vi "Encoder_PanelSim_Global.vi"(0 "menu":T5=enum."set reset", 5 "EncoderIndex":T4, 7 "Value Set":bool, 9 "Numeric Value":dbl format="%#.4f", 11 "error in (no error)":errorcluster, 12 "String Value":string, 13 "Values":T1) -> (10 "Encoder new":T2={"type"="Encoder", "device"="", "name"="", "data"={"<init"=FALSE, ">count"=0.0, ">period"=0.0, "<samples_to_avg"=0, "<offset"=0.0, "<channel_a"=0, "<channel_b"=0}}, 15 "error out":errorcluster)   [LabVIEW 2019]
doc: "This is used to set and get the last motor output values. This is needed for simulation, since we cannot read these values from the hardware.\n\nThis software is licensed. Open the labview\\readme\\WPI Robotics Library Open Source License.txt file for more information."
uses:
  Encoder Update Ops.ctl
  Encoder proto.ctl
  Encoder data protoo.ctl
  <vilib>/Rock Robotics/SystemInterfaces/Encoder/FPGA_EncoderIdx.ctl
  Encoder Values.ctl
panel:
  out "All Values":T2[](array[typedef])
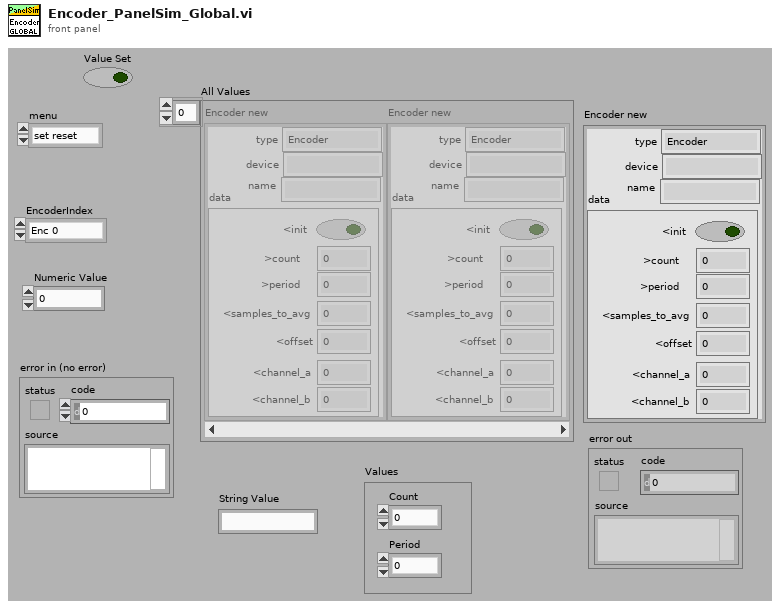
[diagram p1: front panel]
types:
  T1 = typedef "Encoder Values.ctl" = cluster{"Count":dbl, "Period":dbl}
  T2 = typedef "Encoder proto.ctl" = cluster{"type":string, "device":string, "name":string, "data":T3}
  T3 = typedef "Encoder data protoo.ctl" = cluster{"<init":bool, ">count":dbl, ">period":dbl, "<samples_to_avg":i32, "<offset":dbl, "<channel_a":i32, "<channel_b":i32}
  T4 = typedef "FPGA_EncoderIdx.ctl" = enum8{"Enc 0", "Enc 1", "Enc 2", "Enc 3", "Enc 4", "Enc 5", "Enc 6", "Enc 7", "Invalid"}
  T5 = typedef "Encoder Update Ops.ctl" = enum16{"set init", "set count", "set period", "set reset", "set samples_to_avg", "get", "delete", "JSON update", "set name", "transmit initial", "reset", "set channel_a", "set channel_b", "set values"}
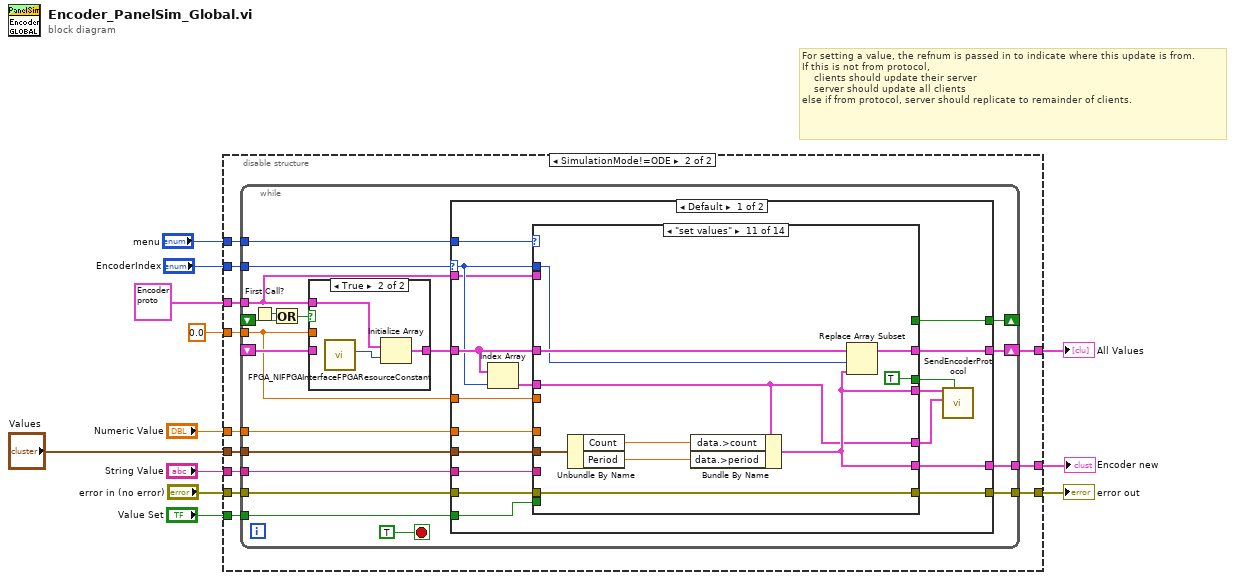
[diagram p0: block diagram]
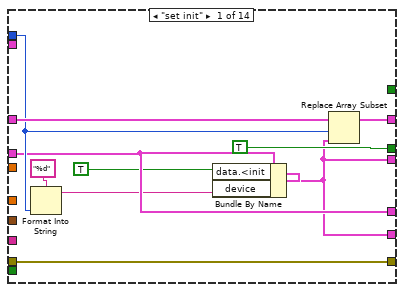
[diagram p3: hidden frame]
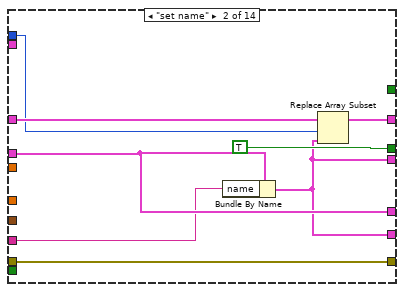
[diagram p4: hidden frame]
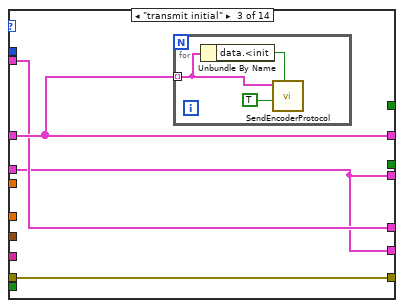
[diagram p5: hidden frame]
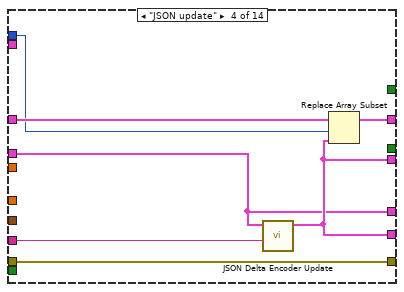
[diagram p6: hidden frame]
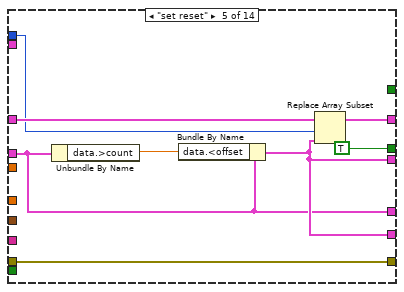
[diagram p7: hidden frame]
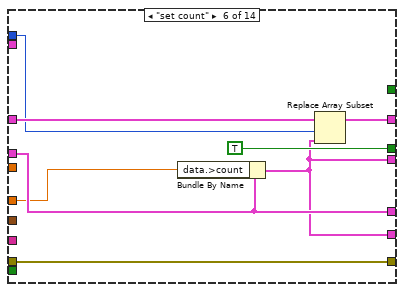
[diagram p8: hidden frame]
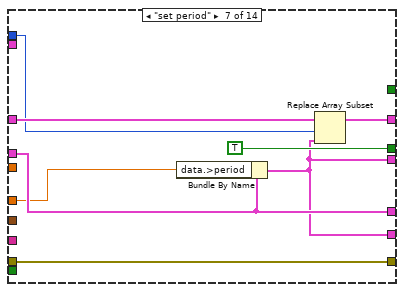
[diagram p9: hidden frame]
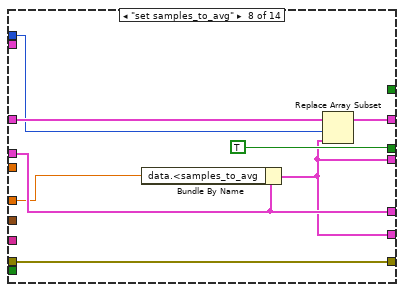
[diagram p10: hidden frame]
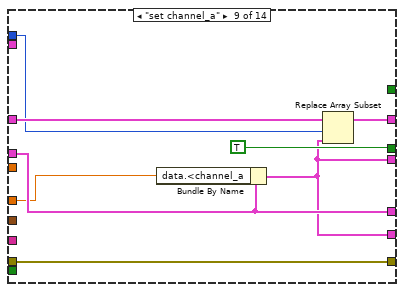
[diagram p11: hidden frame]
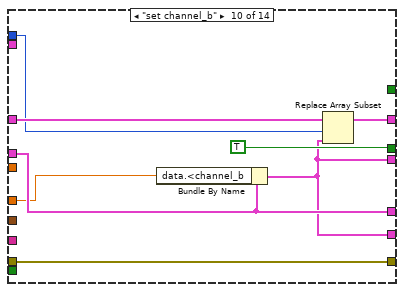
[diagram p12: hidden frame]
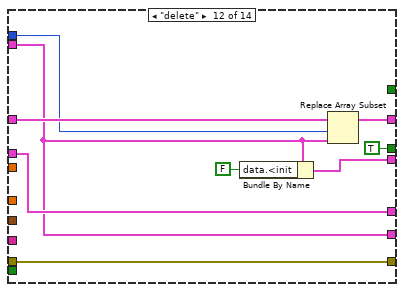
[diagram p13: hidden frame]
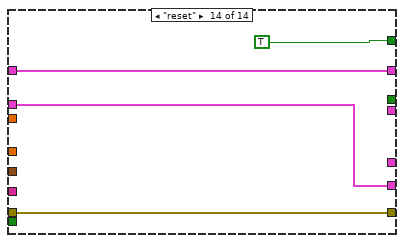
[diagram p15: hidden frame]
diagram:
  # "For setting a value, the refnum is passed in to indicate where this update is from.\nIf this is not from protocol,\n    clients should update their server\n    server should update all clients\nelse if from protocol, server should replicate to remainder of clients."
  n1 = disable-structure shown="SimulationMode!=ODE" {
    disable-tunnel: "menu" -> [_ w26]
    disable-tunnel: [w14 w25] -> w11
    disable-tunnel: "error in (no error)" -> [w14 w24]
    disable-tunnel: [_ w23] -> w9
    disable-tunnel: 0.0 ("Output") -> [_ w22]
    disable-tunnel: "EncoderIndex" -> [_ w21]
    disable-tunnel: [w13 w20] -> w6
    disable-tunnel: T2 {"type"="Encoder", "device"="", "name"="", "data"={"<init"=FALSE, ">count"=0.0, ">period"=0.0, "<samples_to_avg"=0, "<offset"=0.0, "<channel_a"=0, "<channel_b"=0}} ("Encoder new") -> [w13 w19]
    disable-tunnel: "String Value" -> [_ w18]
    disable-tunnel: "Numeric Value" -> [_ w17]
    disable-tunnel: "Value Set" -> [_ w16]
    disable-tunnel: "Values" -> [_ w15]
    frame condition #0 {
    }
    frame condition #1 (active) {
      n2 = while {
        tunnel: w24 -> [w42]
        shift-right: [w45] -> w23
        shift-left: _ -> [w38]
        tunnel: [w44] -> w20
        tunnel: w26 -> [w43]
        tunnel: [w41] -> w25
        tunnel: w21 -> [w36]
        tunnel: w22 -> [w37]
        tunnel: w19 -> [w35]
        tunnel: w18 -> [w34]
        tunnel: w17 -> [w33]
        tunnel: w16 -> [w32]
        shift-right: [w28] -> _
        shift-left: _ -> [w29]
        tunnel: w15 -> [w27]
        stop <- TRUE stop-if-true
        n3 = First Call?() -> (First Call?: T/F=w31:bool)
        n4 = Or(x=w31, y=w29) -> (x .or. y?=w30:bool)
        n5 = case shown="True" w30 {
          tunnel: [w173 w176] -> w39
          tunnel: w38 -> [w173 _]
          tunnel: w37 -> [_ _]
          tunnel: w35 -> [_ w175]
          frame False {
          }
          frame True {
            n6 = call <vilib>:"FPGA_NIFPGAInterfaceFPGAResourceConstant.vi"() -> ("NumberOfEncoders"=w174:u32)  [unwired: 11 out]
            n7 = Initialize Array(w175, w174) -> (w176:T2[])
          }
        }
        n8 = case shown="Default" w36 {
          selector: w36 -> [w56 _]
          tunnel: [w63 w172] -> w45
          tunnel: [w62 w170] -> w44
          tunnel: w43 -> [w61 _]
          tunnel: w42 -> [w60 w171]
          tunnel: [w59 w171] -> w41
          tunnel: w39 -> [w58 w172]
          tunnel: w37 -> [w57 _]
          tunnel: w35 -> [w54 w170]
          tunnel: w34 -> [w53 _]
          tunnel: w33 -> [w52 _]
          tunnel: w32 -> [w48 _]
          tunnel: [w47 _] -> w28
          tunnel: w27 -> [w46 _]
          frame Default {
            n9 = Index Array(array=w58, index=w56) -> (element=w55:T2)
            n10 = case shown="\"set values\"" w61 {
              tunnel: [w73 w81 w84 w95 w103 w111 w119 w127 w135 w143 w153 w161 w165 w169] -> w63
              tunnel: w58 -> [w71 w79 w84 w93 w101 w109 w117 w125 w133 w141 w151 w162 w165 w169]
              tunnel: [w64 w75 w82 w91 w98 w105 w113 w121 w129 w137 w148 w156 w163 w167] -> w62
              tunnel: [w72 w80 w85 w94 w102 w110 w118 w126 w134 w142 w152 w160 w164 w168] -> w59
              tunnel: w60 -> [w72 w80 w85 w94 w102 w110 w118 w126 w134 w142 w152 w160 w164 w168]
              tunnel: w56 -> [w68 w77 _ w92 w99 w107 w115 w123 w131 w139 w149 w157 _ _]
              tunnel: w57 -> [_ _ _ _ _ _ _ _ _ _ _ _ _ _]
              tunnel: [w64 w75 w82 w91 w98 w105 w113 w121 w129 w137 w148 w155 _ _] -> w50
              tunnel: [w67 w76 w83 w89 w97 w106 w114 w122 w130 w138 w144 w158 _ _] -> w49
              tunnel: [TRUE TRUE _ _ TRUE TRUE TRUE TRUE TRUE TRUE TRUE TRUE _ _] -> w51
              tunnel: w55 -> [w67 w76 w82 w89 w97 w106 w114 w122 w130 w138 w144 w158 w163 w167]
              tunnel: w54 -> [_ _ w83 _ _ _ _ _ _ _ _ w156 _ _]
              tunnel: w53 -> [_ w74 _ w90 _ _ _ _ _ _ _ _ _ _]
              tunnel: w52 -> [_ _ _ _ _ w104 w112 w120 w128 w136 _ _ _ _]
              tunnel: w48 -> [_ _ _ _ _ _ _ _ _ _ _ _ _ _]
              tunnel: [_ _ _ _ _ _ _ _ _ _ _ _ _ TRUE] -> w47
              tunnel: w46 -> [_ _ _ _ _ _ _ _ _ _ w147 _ _ _]
              frame "set init" {
                n11 = Format Into String(format string="%d", w68) -> (resulting string=w65:string)  [unwired: 2 in, 1 out]
                n12 = Bundle By Name(cluster=w67, "data.<init"=TRUE, "device"=w65) -> (w64:T2)
                n13 = Replace Array Subset(array=w71, new element=w64, index=w68) -> (w73:T2[])
              }
              frame "set name" {
                n14 = Bundle By Name(cluster=w76, "name"=w74) -> (w75:T2)
                n15 = Replace Array Subset(array=w79, new element=w75, index=w77) -> (w81:T2[])
              }
              frame "transmit initial" {
                n16 = for {
                  tunnel: w84 -> [w86] mode=indexing
                  n17 = Unbundle By Name(w86) -> ("data.<init"=w88:bool)
                  n18 = call "SendEncoderProtocol.vi"("Send"=w88, "Initialize"=TRUE, "Encoder new"=w86) -> ()  [unwired: 9 in]
                }
              }
              frame "JSON update" {
                n19 = call "JSON Delta Encoder Update.vi"("Delta JSON"=w90, "input"=w89) -> ("output"=w91:T2)  [unwired: 8 in, 1 out]
                n20 = Replace Array Subset(array=w93, new element=w91, index=w92) -> (w95:T2[])
              }
              frame "set reset" {
                n21 = Unbundle By Name(w97) -> ("data.>count"=w96:dbl)
                n22 = Bundle By Name(cluster=w97, "data.<offset"=w96) -> (w98:T2)
                n23 = Replace Array Subset(array=w101, new element=w98, index=w99) -> (w103:T2[])
              }
              frame "set count" {
                n24 = Bundle By Name(cluster=w106, "data.>count"=w104) -> (w105:T2)
                n25 = Replace Array Subset(array=w109, new element=w105, index=w107) -> (w111:T2[])
              }
              frame "set period" {
                n26 = Bundle By Name(cluster=w114, "data.>period"=w112) -> (w113:T2)
                n27 = Replace Array Subset(array=w117, new element=w113, index=w115) -> (w119:T2[])
              }
              frame "set samples_to_avg" {
                n28 = Bundle By Name(cluster=w122, "data.<samples_to_avg"=w120) -> (w121:T2)
                n29 = Replace Array Subset(array=w125, new element=w121, index=w123) -> (w127:T2[])
              }
              frame "set channel_a" {
                n30 = Bundle By Name(cluster=w130, "data.<channel_a"=w128) -> (w129:T2)
                n31 = Replace Array Subset(array=w133, new element=w129, index=w131) -> (w135:T2[])
              }
              frame "set channel_b" {
                n32 = Bundle By Name(cluster=w138, "data.<channel_b"=w136) -> (w137:T2)
                n33 = Replace Array Subset(array=w141, new element=w137, index=w139) -> (w143:T2[])
              }
              frame "set values" {
                n34 = Unbundle By Name(w147) -> ("Count"=w146:dbl, "Period"=w145:dbl)
                n35 = Bundle By Name(cluster=w144, "data.>count"=w146, "data.>period"=w145) -> (w148:T2)
                n36 = Replace Array Subset(array=w151, new element=w148, index=w149) -> (w153:T2[])
              }
              frame "delete" {
                n37 = Bundle By Name(cluster=w156, "data.<init"=FALSE) -> (w155:T2)
                n38 = Replace Array Subset(array=w162, new element=w156, index=w157) -> (w161:T2[])
              }
              frame "get" {
              }
              frame "reset" {
              }
            }
            n39 = call "SendEncoderProtocol.vi"("Send"=w51, "Encoder old"=w49, "Encoder new"=w50) -> ()  [unwired: 9 in]
          }
          frame "Invalid" {
            # "Do nothing if \nchannel is Invalid."
          }
        }
      }
    }
  }
  "error out" <- w11
  "All Values" <- w9
  "Encoder new" <- w6
